vi "Peter.vi"(9 "REPL":string, 10 "Send":string) -> ()   [LabVIEW 2020]
panel:
  in  "start pybricks":bool
  out "Cover":bool
  in  "Script":string
  in  "Buffer":string
  in  "Disconnect":bool
  in  "EV3":T1={"EV3 IP Address"="192.168.7.116", "Username"="robot", "password"="maker"}
  in  "Help":bool
  in  "Connect":bool
  in  "Stop Button":bool
  out "Running Script":bool
  in  "Abort":bool
  in  "xPort":string
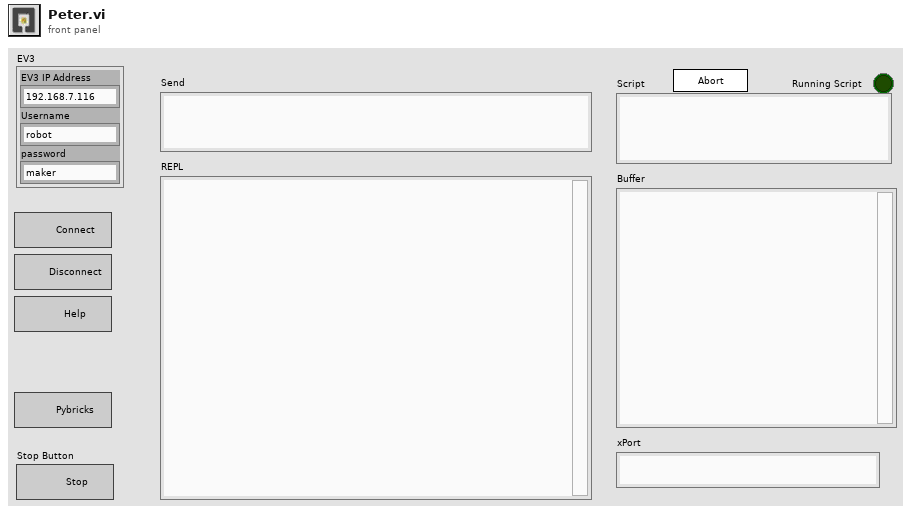
[diagram p1: front panel]
types:
  T1 = cluster{"EV3 IP Address":string, "Username":string, "password":string}
  T2 = enum32{"Invalid", "Standard", "Closed", "Hidden", "Minimized", "Maximized"}
  T3 = typedef "eventvkey.ctl" = enum16{"ASCII", "Enter", "Return", "Shift", "Ctrl", "Alt", "Cmd", "Opt", "Caps", "NumLock", "Clear", "Break", "Up", "Down", "Left", "Right", "Insert", "Delete", "Home", "End", "PageUp", "PageDown", "Escape", "Help", "Pause", "ScrollLock", "F1", "F2", "F3", "F4", "F5", "F6", "F7", "F8", "F9", "F10", "F11", "F12", "F13", "F14", "F15", "F16", "F17", "F18", "F19", "F20", "F21", "F22", "F23", "F24", "Play", "VolumeUp", "VolumeDown", "Mute", "Two Byte Char"}
  T4 = cluster{"Shift":bool, "Ctrl":bool, "Alt":bool, "Cmd":bool, "Opt":bool}
  T5 = cluster{"Char":i16, "VKey":T3, "PlatMods":cluster{"Shift":bool, "Ctrl":bool, "Alt":bool, "Cmd":bool, "Opt":bool}}
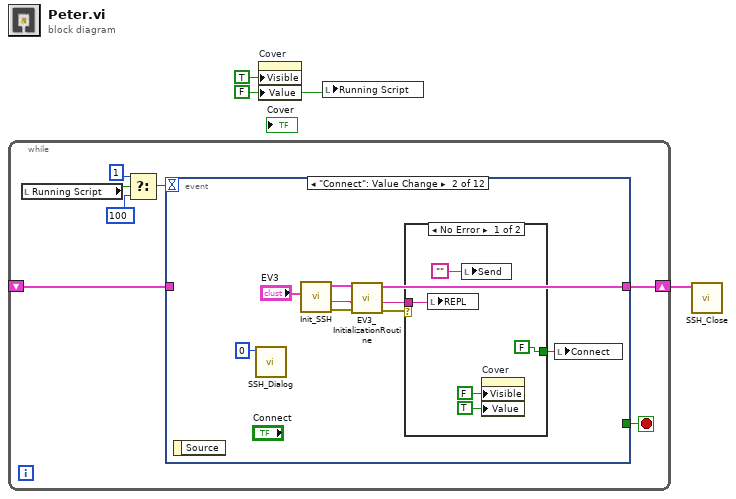
[diagram p0: block diagram]
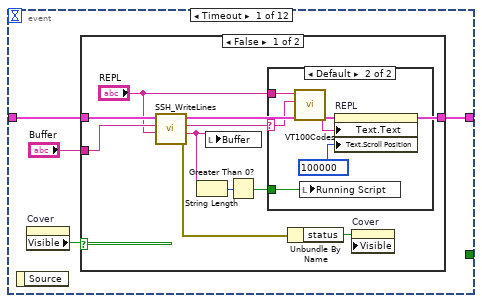
[diagram p2: hidden frame]
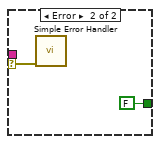
[diagram p5: hidden frame]
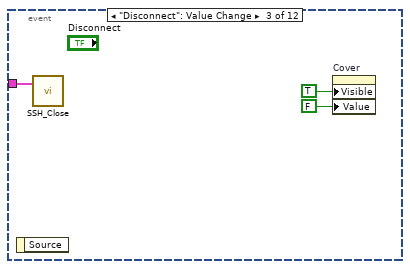
[diagram p6: hidden frame]
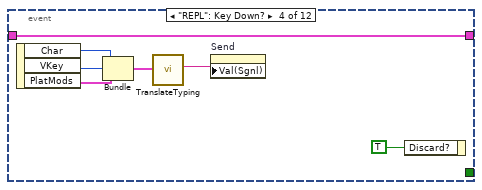
[diagram p7: hidden frame]
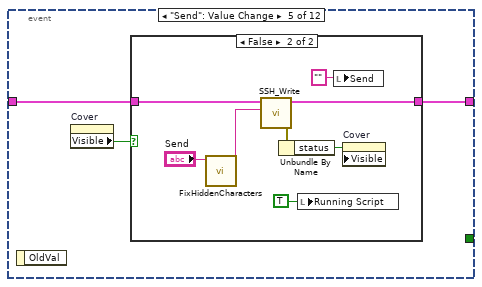
[diagram p8: hidden frame]
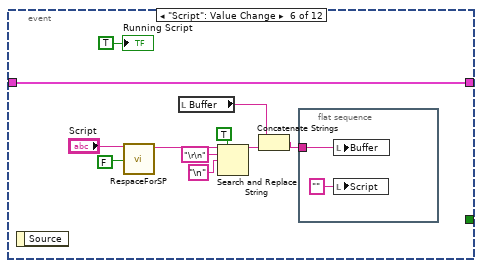
[diagram p10: hidden frame]
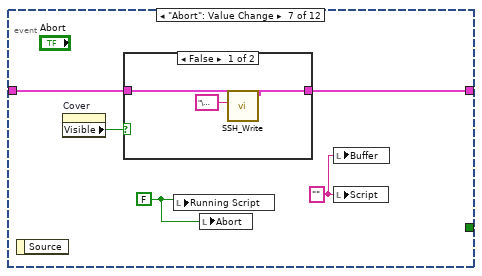
[diagram p11: hidden frame]
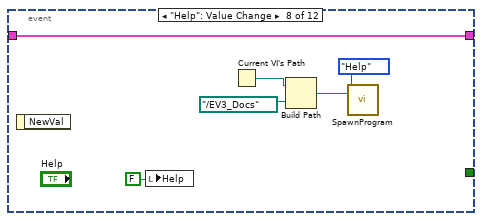
[diagram p13: hidden frame]
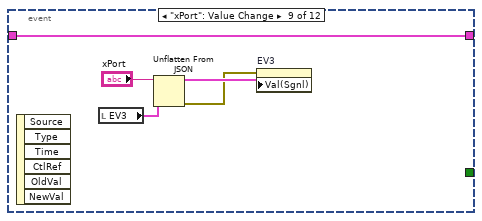
[diagram p14: hidden frame]
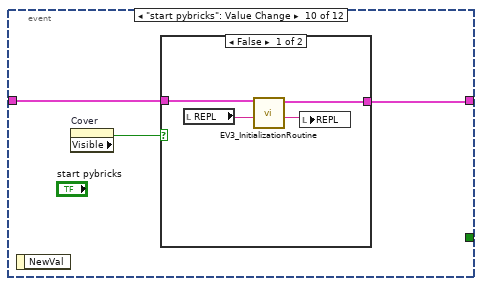
[diagram p15: hidden frame]
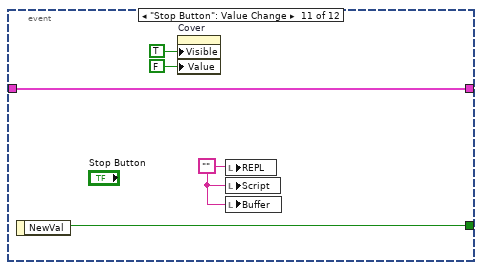
[diagram p17: hidden frame]
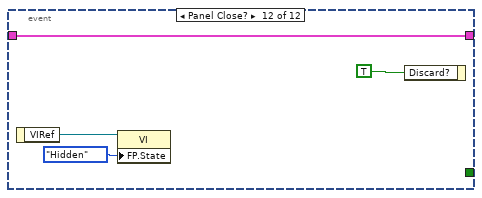
[diagram p18: hidden frame]
diagram:
  w1 = FALSE ("Cover")
  n1 = while {
    shift-right: [w9] -> w2
    shift-left: _ -> [w8]
    stop <- w10 stop-if-true
    n2 = local read "Running Script"() -> (w4:bool)
    n3 = Select(t=1, s=w4, f=100) -> (s? t:f=w5:i32)
    n4 = event shown="[1] \"Connect\": Value Change" {
      selector: _ -> [_ _ _ _ _ _ _ _ _ _ _ _]
      dyn-events: _ -> [_ _ _ _ _ _ _ _ _ _ _ _]
      timeout: w5 -> [_ _ _ _ _ _ _ _ _ _ _ _]
      tunnel: [_ _ _ _ _ _ _ _ _ _ w113 _] -> w10
      tunnel: [w14 w37 _ w55 w58 w79 w84 w96 w101 w102 w114 w118] -> w9
      tunnel: w8 -> [w12 _ w49 w55 w59 w79 w85 w96 w101 w103 w114 w118]
      event Timeout {
        n5 = event-data() -> ()  [unwired: 1 in, 1 out]
        n6 = property on="Cover" class="Bool (strict)"() -> ("Visible"=w13:bool)  [unwired: 2 in, 2 out]
        n7 = case shown="False" w13 {
          tunnel: [w21 w30] -> w14
          tunnel: w12 -> [w24 w30]
          tunnel: "Buffer" -> [w23 _]
          frame False {
            n8 = call "SSH_WriteLines.vi"("REPL"="REPL", "Buffer"=w23, "Python in"=w24) -> ("error out"=w18:errorcluster, "Rest"=w16:string, "Reply"=w20:string, "Python out"=w21:cluster{"Python":refnum<k35>, "py file":path})  [unwired: 5 in]
            n9 = String Length(string=w16) -> (length=w17:i32)
            n10 = local write "Buffer"(w16) -> ()
            n11 = Greater Than 0?(x=w17) -> (x > 0?=w15:bool)
            n12 = case shown="Default" w20 {
              selector: w20 -> [_ w26]
              tunnel: "REPL" -> [_ w27]
              tunnel: w15 -> [_ w25]
              frame "" {
              }
              frame Default {
                n13 = call "VT100Codes.vi"("read buffer"=w26, "Console In"=w27) -> ("Console Out"=w28:string)  [unwired: 9 in]
                n14 = local write "Running Script"(w25) -> ()
                n15 = property on="REPL" class="Str"("Text.Text"=w28, "Text.Scroll Position"=u32 100000 ("Text.Selection:Start")) -> ()  [unwired: 2 in, 2 out]
              }
            }
            n16 = Unbundle By Name(w18) -> ("status"=w22:bool)
            n17 = property on="Cover" class="Bool (strict)"("Visible"=w22) -> ()  [unwired: 2 in, 2 out]
          }
          frame True {
          }
        }
      }
      event "Connect": Value Change {
        n18 = event-data() -> ()  [unwired: 1 in, 1 out]
        n19 = call "SSH_Dialog.vi"("Slide"=u8 0) -> ()  [unwired: 11 in]
        n20 = call "Init_SSH.vi"("EV3"="EV3") -> ("error out"=w38:errorcluster, "Console out"=w33:string, "Python out"=w39:cluster{"Python":refnum<k35>, "py file":path})  [unwired: 8 in]
        n21 = call "EV3_InitializationRoutine.vi"("error in (no error)"=w38, "Console In"=w33, "Python in"=w39) -> ("error out"=w36:errorcluster, "Console Out"=w32:string, "Python out"=w37:cluster{"Python":refnum<k35>, "py file":path})  [unwired: 6 in]
        n22 = case shown="No Error" w36 {
          selector: w36 -> [_ w46]
          tunnel: w32 -> [w41 _]
          tunnel: [FALSE ("Cover") FALSE ("Cover")] -> w31
          frame No Error {
            n23 = local write "REPL"(w41) -> ()
            n24 = local write "Send"("") -> ()
            n25 = property on="Cover" class="Bool (strict)"("Visible"=FALSE, "Value"=TRUE ("Cover")) -> ()  [unwired: 2 in, 2 out]
          }
          frame Error {
            n26 = call <vilib>:"Simple Error Handler.vi"("error in (no error)"=w46) -> ()  [unwired: 4 in, 5 out]
          }
        }
        n27 = local write "Connect"(w31) -> ()
      }
      event "Disconnect": Value Change {
        n28 = event-data() -> ()  [unwired: 1 in, 1 out]
        n29 = call "SSH_Close.vi"("Python in"=w49) -> ()  [unwired: 11 in]
        n30 = property on="Cover" class="Bool (strict)"("Visible"=TRUE, "Value"=FALSE ("Cover")) -> ()  [unwired: 2 in, 2 out]
      }
      event "REPL": Key Down? {
        n31 = event-data() -> ("Char"=w53:i16, "VKey"=w52:T3, "PlatMods"=w51:T4)  [unwired: 1 in]
        n32 = Bundle("Char"=w53, "VKey"=w52, "PlatMods"=w51) -> (w54:T5)  [unwired: 1 in]
        n33 = call "TranslateTyping.vi"("Cluster"=w54) -> ("key"=w50:string)  [unwired: 10 in]
        n34 = property on="Send" class="Str"("Val(Sgnl)"=w50) -> ()  [unwired: 2 in, 2 out]
        n35 = event-data("Discard?"=TRUE) -> ()  [unwired: 1 in, 1 out]
      }
      event "Send": Value Change {
        n36 = event-data() -> ()  [unwired: 1 in, 1 out]
        n37 = property on="Cover" class="Bool (strict)"() -> ("Visible"=w57:bool)  [unwired: 2 in, 2 out]
        n38 = case shown="False" w57 {
          tunnel: w59 -> [w60 w66]
          tunnel: [w60 w65] -> w58
          frame True {
          }
          frame False {
            n39 = call "FixHiddenCharacters.vi"("String in"="Send") -> ("String out"=w62:string)  [unwired: 10 in]
            n40 = call "SSH_Write.vi"("Text to write"=w62, "Python in"=w66) -> ("error out"=w64:errorcluster, "Python out"=w65:cluster{"Python":refnum<k35>, "py file":path})  [unwired: 8 in]
            n41 = Unbundle By Name(w64) -> ("status"=w67:bool)
            n42 = local write "Running Script"(TRUE ("Running Script")) -> ()
            n43 = local write "Send"("" ("Write text")) -> ()
            n44 = property on="Cover" class="Bool (strict)"("Visible"=w67) -> ()  [unwired: 2 in, 2 out]
          }
        }
      }
      event "Script": Value Change {
        n45 = event-data() -> ()  [unwired: 1 in, 1 out]
        n46 = call "RespaceForSP.vi"("Keep spaces?"=FALSE, "Code"="Script") -> ("Cleaned for SPIKE"=w74:string)  [unwired: 9 in]
        n47 = local read "Buffer"() -> (w71:string)
        n48 = Search and Replace String(replace all?=TRUE ("replace all? (F)"), input string=w74, search string="\r\n", replace string="\n" ("search string")) -> (result string=w70:string)  [unwired: 4 in, 3 out]
        n49 = Concatenate Strings(w71, w70) -> (w69:string)
        n50 = flat-sequence {
          tunnel: w69 -> [w81]
          frame #0 {
            n51 = local write "Buffer"(w81) -> ()
            n52 = local write "Script"("" ("Script")) -> ()
          }
        }
        "Running Script" <- TRUE ("Running Script")
      }
      event "Abort": Value Change {
        w86 = "" ("Script")
        w83 = FALSE ("Running Script")
        n53 = event-data() -> ()  [unwired: 1 in, 1 out]
        n54 = property on="Cover" class="Bool (strict)"() -> ("Visible"=w82:bool)  [unwired: 2 in, 2 out]
        n55 = case shown="False" w82 {
          tunnel: w85 -> [w89 w90]
          tunnel: [w88 w90] -> w84
          frame False {
            n56 = call "SSH_Write.vi"("Text to write"="\u0003", "Python in"=w89) -> ("Python out"=w88:cluster{"Python":refnum<k35>, "py file":path})  [unwired: 8 in, 1 out]
          }
          frame True {
          }
        }
        n57 = local write "Running Script"(w83) -> ()
        n58 = local write "Abort"(w83) -> ()
        n59 = local write "Buffer"(w86) -> ()
        n60 = local write "Script"(w86) -> ()
      }
      event "Help": Value Change {
        n61 = event-data() -> ()  [unwired: 1 in, 1 out]
        n62 = local write "Help"(FALSE ("Help")) -> ()
        n63 = Current VI's Path() -> (path=w94:path)
        n64 = Build Path(base path=w94, name or relative path=path "../EV3_Docs") -> (appended path=w91:path)
        n65 = call "SpawnProgram.vi"("Server"=w91, "Dialog"=enum16{"Help", "Files"}."Help") -> ()  [unwired: 10 in]
      }
      event "xPort": Value Change {
        n66 = event-data() -> ()  [unwired: 1 in, 6 out]
        n67 = local read "EV3"() -> (w97:T1)
        n68 = Unflatten From JSON(JSON string="xPort", type and defaults=w97) -> (value=w99:T1, error out=w98:errorcluster)  [unwired: 5 in]
        n69 = property on="EV3" class="Clust (strict)"(error in=w98, "Val(Sgnl)"=w99) -> ()  [unwired: 1 in, 2 out]
      }
      event "start pybricks": Value Change {
        n70 = event-data() -> ()  [unwired: 1 in, 1 out]
        n71 = property on="Cover" class="Bool (strict)"() -> ("Visible"=w104:bool)  [unwired: 2 in, 2 out]
        n72 = case shown="False" w104 {
          tunnel: w103 -> [w107 w109]
          tunnel: [w108 w109] -> w102
          frame False {
            n73 = local read "REPL"() -> (w106:string)
            n74 = call "EV3_InitializationRoutine.vi"("Console In"=w106, "Python in"=w107) -> ("Console Out"=w105:string, "Python out"=w108:cluster{"Python":refnum<k35>, "py file":path})  [unwired: 7 in, 1 out]
            n75 = local write "REPL"(w105) -> ()
          }
          frame True {
          }
        }
      }
      event "Stop Button": Value Change {
        w110 = ""
        n76 = event-data() -> ("NewVal"=w113:bool)  [unwired: 1 in]
        n77 = property on="Cover" class="Bool (strict)"("Visible"=TRUE, "Value"=FALSE ("Cover")) -> ()  [unwired: 2 in, 2 out]
        n78 = local write "REPL"(w110) -> ()
        n79 = local write "Script"(w110) -> ()
        n80 = local write "Buffer"(w110) -> ()
      }
      event Panel Close? {
        n81 = event-data() -> ("VIRef"=w116:refnum<vi>)  [unwired: 1 in]
        n82 = property class="VI"(reference=w116, "FP.State"=T2."Hidden" ("Front Panel Window:State")) -> ()  [unwired: 1 in, 2 out]
        n83 = event-data("Discard?"=TRUE) -> ()  [unwired: 1 in, 1 out]
      }
    }
  }
  n84 = property on="Cover" class="Bool (strict)"("Visible"=TRUE, "Value"=w1) -> ()  [unwired: 2 in, 2 out]
  n85 = local write "Running Script"(w1) -> ()
  n86 = call "SSH_Close.vi"("Python in"=w2) -> ()  [unwired: 11 in]
